vi "Water Temperature-Depth Control.vi"(4 "State":i16, 5 "Time":dbl format="%.2f", 6 "Sensor Values":dbl[](array[numeric]), 7 "Set Points":dbl[](array[numeric])) -> (0 "required data":T1={"Set Point names"=["Hot=1 Cold=0", "full height"], "required number of setpoints"=2, "required number of sensors"=3, "Sensor names"=["Water depth", "Water temperature", "Air temperature"]}, 3 "output value":dbl)   [LabVIEW 2012]
panel:
  # "Enter the correct information for this control code in the required data structure below. Then make the current value default by right clicking on the border of the data structure. Select \"data operations\" and then select \"make current value default\". These values will be displayed by process controller."
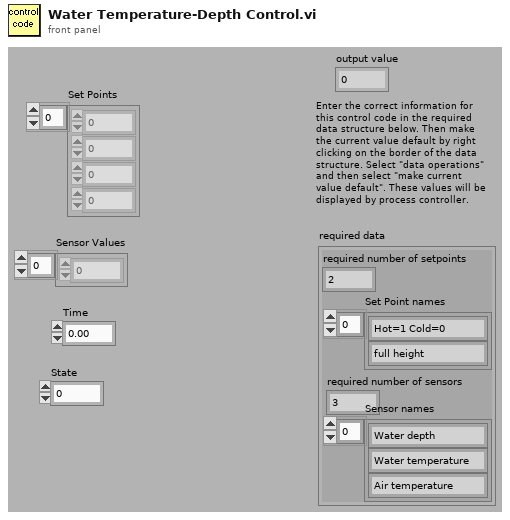
[diagram p1: front panel]
types:
  T1 = cluster{"Set Point names":string[], "required number of setpoints":u8, "required number of sensors":u8, "Sensor names":string[]}
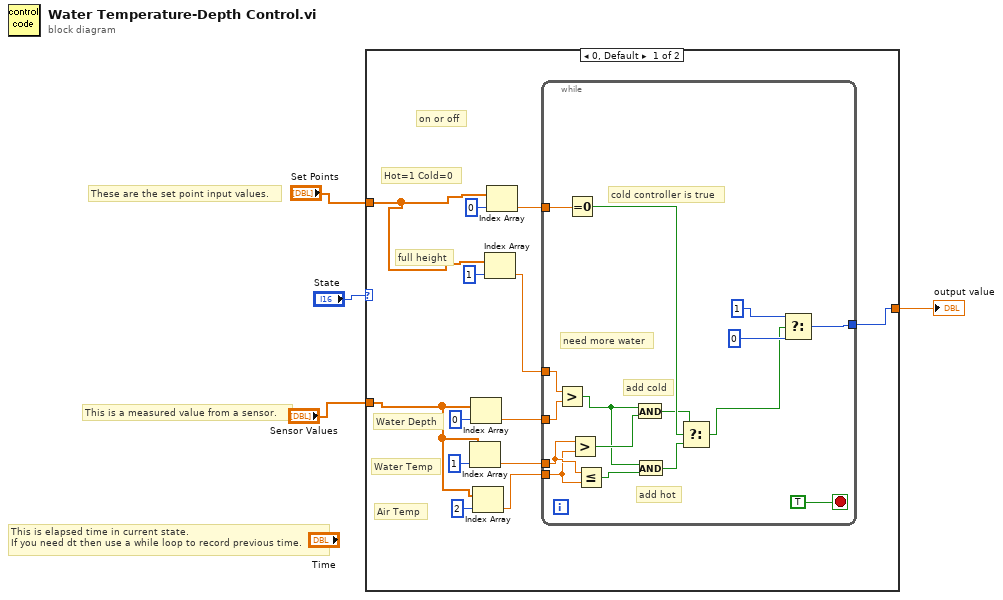
[diagram p0: block diagram]
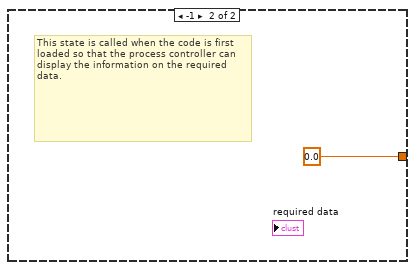
[diagram p2: hidden frame]
diagram:
  # "These are the set point input values."
  # "This is a measured value from a sensor."
  # "This is elapsed time in current state.\nIf you need dt then use a while loop to record previous time."
  n1 = case shown="0, Default" "State" {
    tunnel: [w17 0.0 ("fraction on")] -> w3
    tunnel: "Set Points" -> [w7 _]
    tunnel: "Sensor Values" -> [w11 _]
    frame 0, Default {
      # "full height"
      # "Air Temp"
      # "Water Temp"
      # "on or off"
      # "Water Depth"
      # "Hot=1 Cold=0"
      n2 = Index Array(array=w11, index=1) -> (element=w10:dbl)
      n3 = Index Array(array=w11, index=0) -> (element=w15:dbl)
      n4 = Index Array(array=w11, index=2) -> (element=w9:dbl)
      n5 = Index Array(array=w7, index=1) -> (element=w6:dbl)
      n6 = Index Array(array=w7, index=0) -> (element=w5:dbl)
      n7 = while {
        tunnel: w6 -> [w32]
        tunnel: [w31] -> w17
        tunnel: w15 -> [w30]
        tunnel: w10 -> [w26]
        tunnel: w9 -> [w25]
        tunnel: w5 -> [w22]
        stop <- TRUE stop-if-true
        # "cold controller is true"
        # "add cold"
        # "add hot"
        # "need more water"
        n8 = Greater?(x=w32, y=w30) -> (0:w23:bool)
        n9 = Equal To 0?(x=w22) -> (x = 0?=w21:bool)
        n10 = Greater?(x=w26, y=w25) -> (0:w29:bool)
        n11 = Less Or Equal?(x=w26, y=w25) -> (x <= y?=w24:bool)
        n12 = And(x=w23, y=w29) -> (x .and. y?=w20:bool)
        n13 = And(x=w23, y=w24) -> (x .and. y?=w19:bool)
        n14 = Select(t=w20, s=w21, f=w19) -> (s? t:f=w18:bool)
        n15 = Select(t=1, s=w18, f=0) -> (s? t:f=w31:i32)
      }
    }
    frame -1 {
      # "This state is called when the code is first loaded so that the process controller can display the information on the required data."
    }
  }
  "output value" <- w3
